vi "FeedbackDecode_FindCamInterface.vi"(2 "ErrorIn":errorcluster) -> (0 "ErrorOut":errorcluster, 1 "CamInterface":string)   [LabVIEW 2020]
uses:
  <vilib>/vision/driver/NI_Vision_Acquisition_Software.lvlib
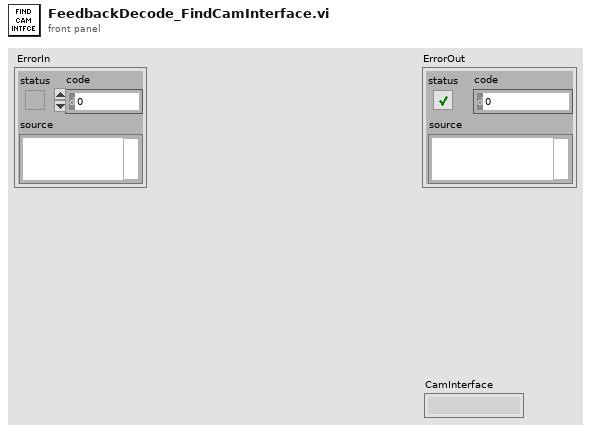
[diagram p1: front panel]
types:
  T1 = cluster{"Type":u32, "Version":u32, "Flags":u32, "SerialNumberHigh":u32, "SerialNumberLow":u32, "BusType":u32, "InterfaceName":string, "VendorName":string, "ModelName":string, "CameraFileName":string, "CameraAttributeURL":string}[]
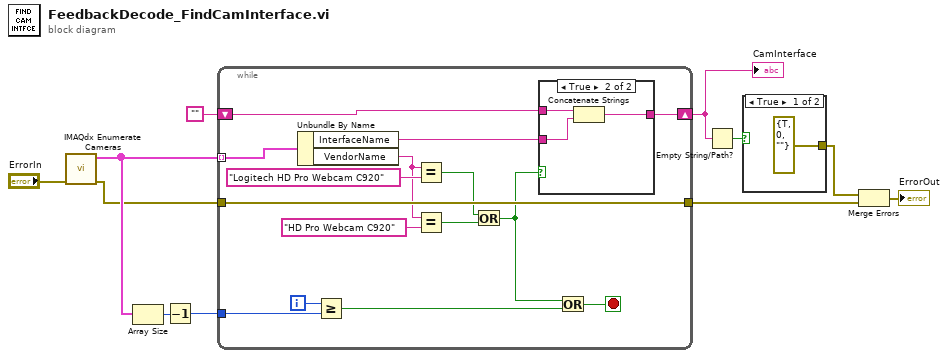
[diagram p0: block diagram]
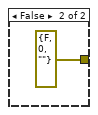
[diagram p2: hidden frame]
diagram:
  n1 = call <vilib>:"IMAQdx Enumerate Cameras.vi"("error in"="ErrorIn") -> ("error out"=w6:errorcluster, "Camera Information Array"=w10:T1)  [unwired: 9 in]
  n2 = Array Size(array=w10) -> (size(s)=w9:i32)
  n3 = Decrement(x=w9) -> (x-1=w8:i32)
  n4 = while {
    tunnel: w10 -> [w26] mode=indexing
    shift-right: [w22] -> w5
    shift-left: "" -> [w23]
    tunnel: w8 -> [w21]
    tunnel: w6 -> [w17]
    tunnel: [w17] -> w2
    i -> [w20]
    stop <- w18 stop-if-true
    n5 = Unbundle By Name(w26) -> ("InterfaceName"=w24:string, "VendorName"=w15:string)
    n6 = Greater Or Equal?(x=w20, y=w21) -> (x >= y?=w19:bool)
    n7 = Equal?(x=w15, y="Logitech HD Pro Webcam C920") -> (x = y?=w13:bool)
    n8 = Equal?(x=w15, y="HD Pro Webcam C920") -> (x = y?=w14:bool)
    n9 = Or(x=w13, y=w14) -> (x .or. y?=w12:bool)
    n10 = case shown="True" w12 {
      tunnel: w24 -> [_ w29]
      tunnel: w23 -> [w27 w30]
      tunnel: [w27 w28] -> w22
      frame False {
      }
      frame True {
        n11 = Concatenate Strings(w30, w29) -> (w28:string)
      }
    }
    n12 = Or(x=w12, y=w19) -> (x .or. y?=w18:bool)
  }
  "CamInterface" <- w5
  n13 = Empty String/Path?(string/path=w5) -> (empty?=w4:bool)
  n14 = case shown="True" w4 {
    tunnel: [errorcluster {"status"=TRUE, "code"=0, "source"=""} ("error constant") errorcluster {"status"=FALSE, "code"=0, "source"=""} ("error constant")] -> w3
    frame True {
    }
    frame False {
    }
  }
  n15 = Merge Errors(w3, w2) -> (→"ErrorOut":errorcluster)
